vi "BRig_FPGA_v3,91.vi"() -> ()   [LabVIEW 2014]
uses:
  <vilib>/rvi/Emulation/niFpgaGetClockAttributes.vi
  <vilib>/rvi/Emulation/niFpgaSctlEmulationGetInTimedLoop.vi
  <vilib>/rvi/Emulation/niFpgaEmulationReportErrorSimple.vi
  <vilib>/rvi/eio/common/nirviEmuTemplateMethod_errors.vi
  <vilib>/rvi/Emulation/niFpgaCriticalErrorInLSC.vi
  <vilib>/eio/EIONode/EIONode.xnode
panel:
  in  "L2Led_ON":bool
  in  "L1Led_ON":bool
  in  "Rising(F)_or_Falling(T)":bool
  in  "Solenoid_trig_R":bool
  in  "Solenoid_trig_L":bool
  in  "Solenoid_nTotal_R":u32=100
  in  "Solenoid_nTotal_L":u32=100
  in  "L2Led_Baseline":bool
  in  "L1Led_Baseline":bool
  in  "CueLed_Baseline":bool
  in  "I_allReward":bool
  in  "AnaOut_1":u16
  in  "CueLed_Event":bool
  in  "CueLed_nValley":u32=100
  in  "CueLed_nPeak":u32=100
  in  "LC_Event_l2":bool
  in  "LC_Laser_l2":bool
  in  "LC_nShutter_l2":u32=100
  in  "LC_nValley_l2":u32=100
  in  "LC_nPeak_l2":u32=100
  in  "LR_wrong_nDelay_l2":u32
  in  "LR_reward_nDelay_l2":u32
  in  "LR_wrong_nTotal_l2":u32=100
  in  "LR_reward_nTotal_l2":u32=100
  in  "LR_wrong_laser_l2":bool
  in  "LR_wrong_Event_l2":bool
  in  "LR_reward_Laser_l2":bool
  in  "LR_reward_Event_l2":bool
  out "AnaIn_1":u16
  out "AnaIn_0":u16
  out "timeTrial_count":u32
  in  "timeTrial_trig":bool
  in  "k1__counter_per_ms":u16=100 min=100 max=40000 step=1
  in  "LC_nShutter_l1":u32=100
  in  "AnaOut_0":u16
  in  "LC_nValley_l1":u32=100
  in  "LC_nPeak_l1":u32=100
  in  "LC_Event_l1":bool
  in  "LR_wrong_nTotal_l1":u32=100
  in  "LR_wrong_nDelay_l1":u32
  in  "LR_reward_nTotal_l1":u32=100
  in  "LR_reward_nDelay_l1":u32
  in  "LR_reward_Event_l1":bool
  in  "LR_wrong_Event_l1":bool
  out "SelectWrong":bool
  out "SelectReward":bool
  in  "LR_wrong_Laser_l1":bool
  in  "LR_reward_Laser_l1":bool
  in  "Left(F)_or_Right(T)":bool
  in  "ignoreWrong":bool
  in  "SelectionState":bool
  in  "LC_Laser_l1":bool
  in  "FPGA_Stop":bool
  in  "audioTrigger_L":bool
  in  "audioTrigger_R":bool
  in  "audioFreq_L_kHz":u8=14 min=1 max=14 step=1
  in  "audioAmp_L":u16=1 min=1 max=32767 step=1
  in  "audioFreq_R_kHz":u8=14 min=1 max=14 step=1
  in  "audioAmp_R":u16=1 min=1 max=32767 step=1
  in  "A3_SL":bool
  in  "A1_SR":bool
  in  "Counts_Reset":bool
  out "A4_LickR":u32
  out "A2_LickL":u32
  in  "A6_Act":bool
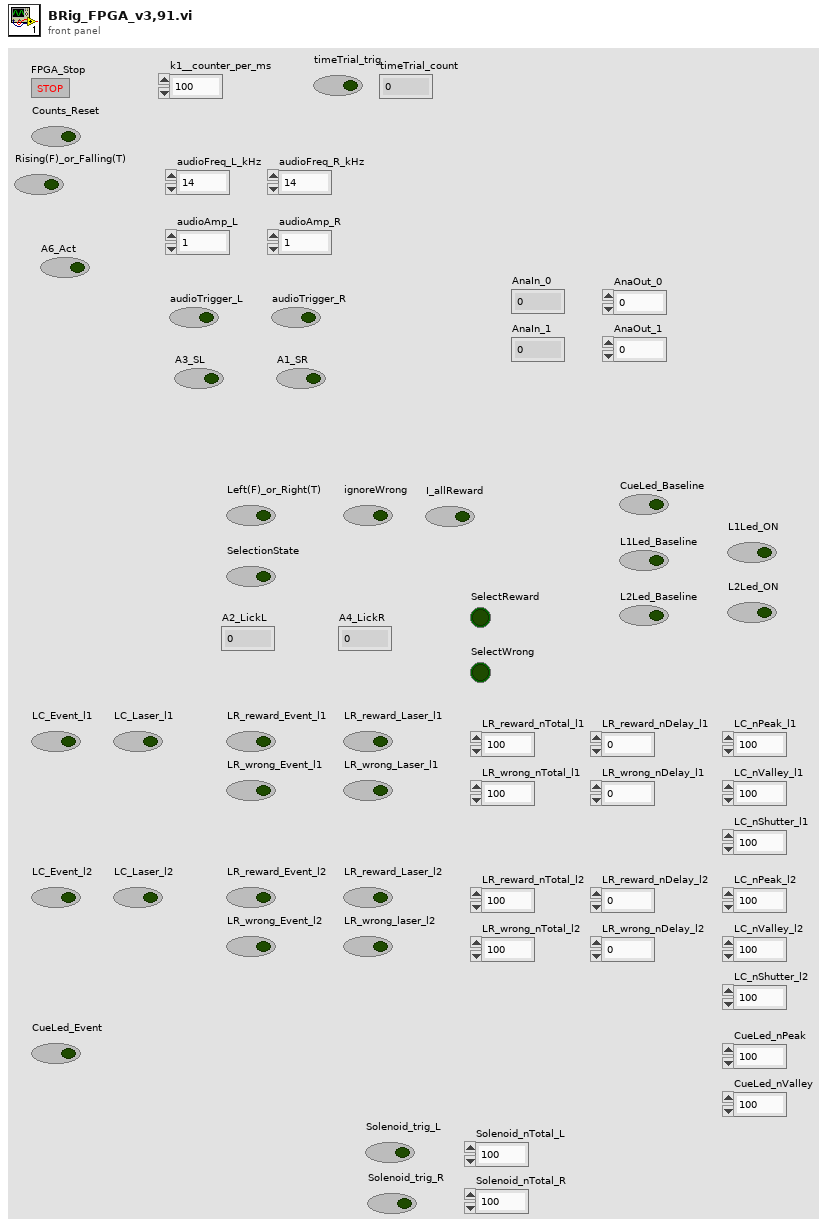
[diagram p1: front panel]
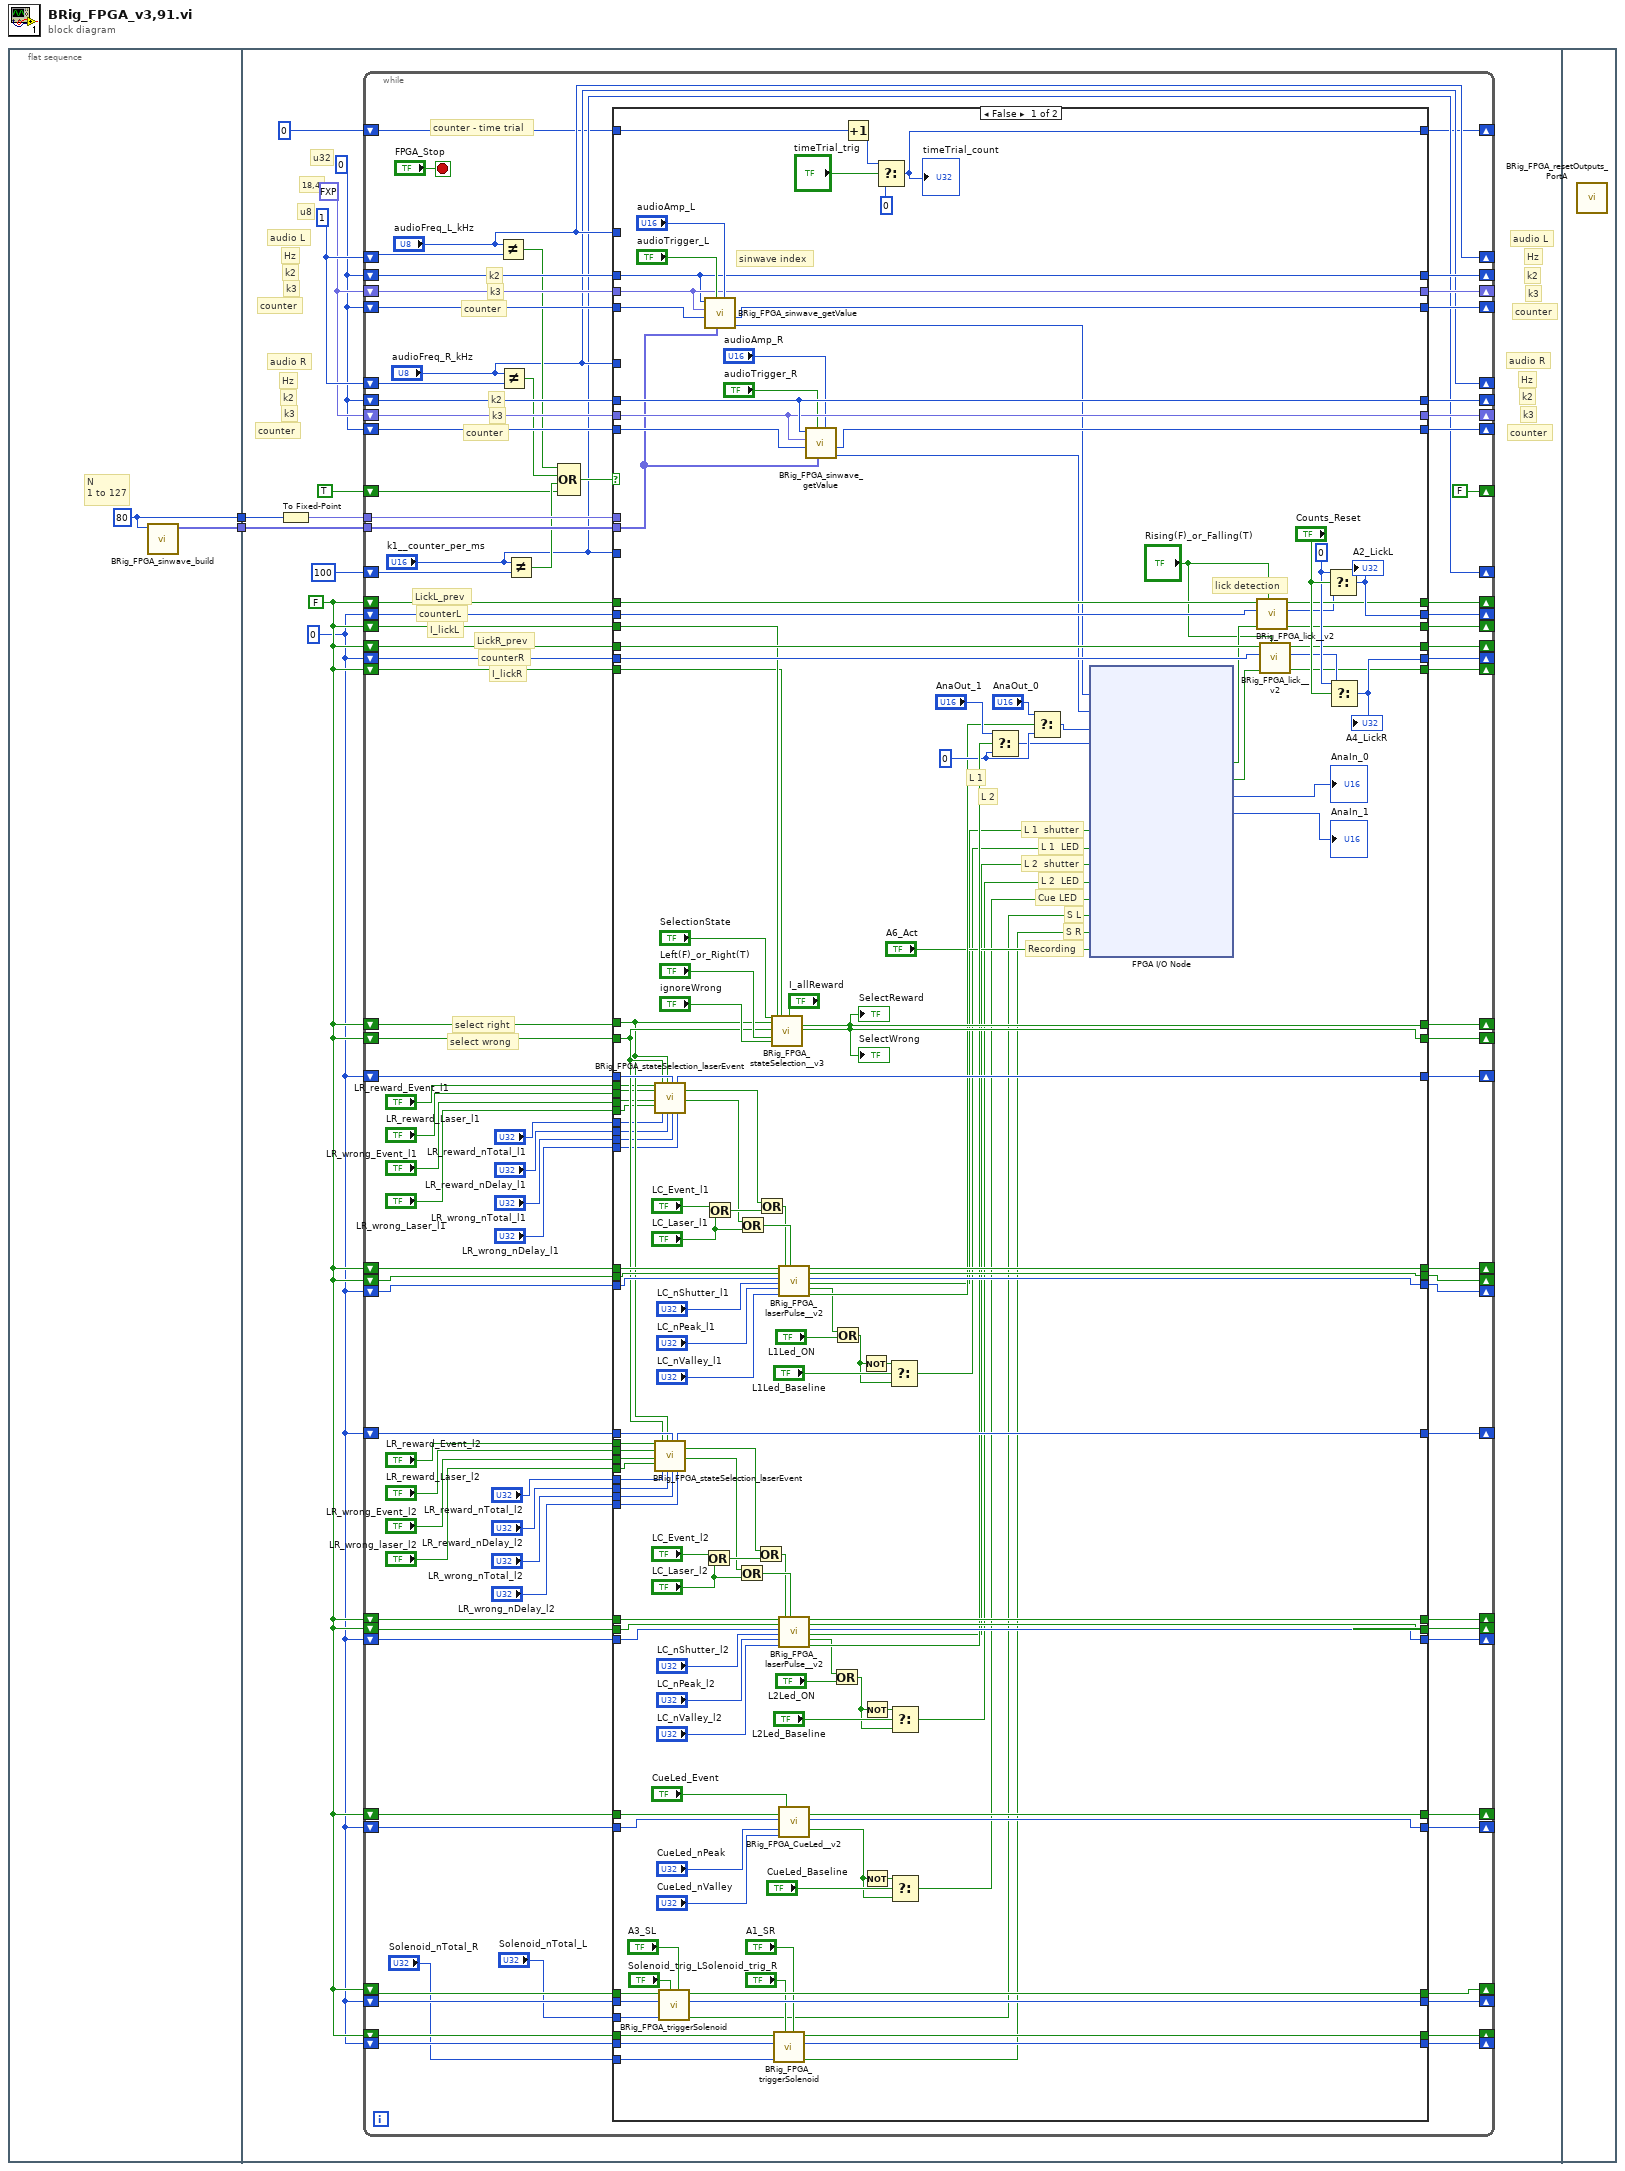
[diagram p0: block diagram]
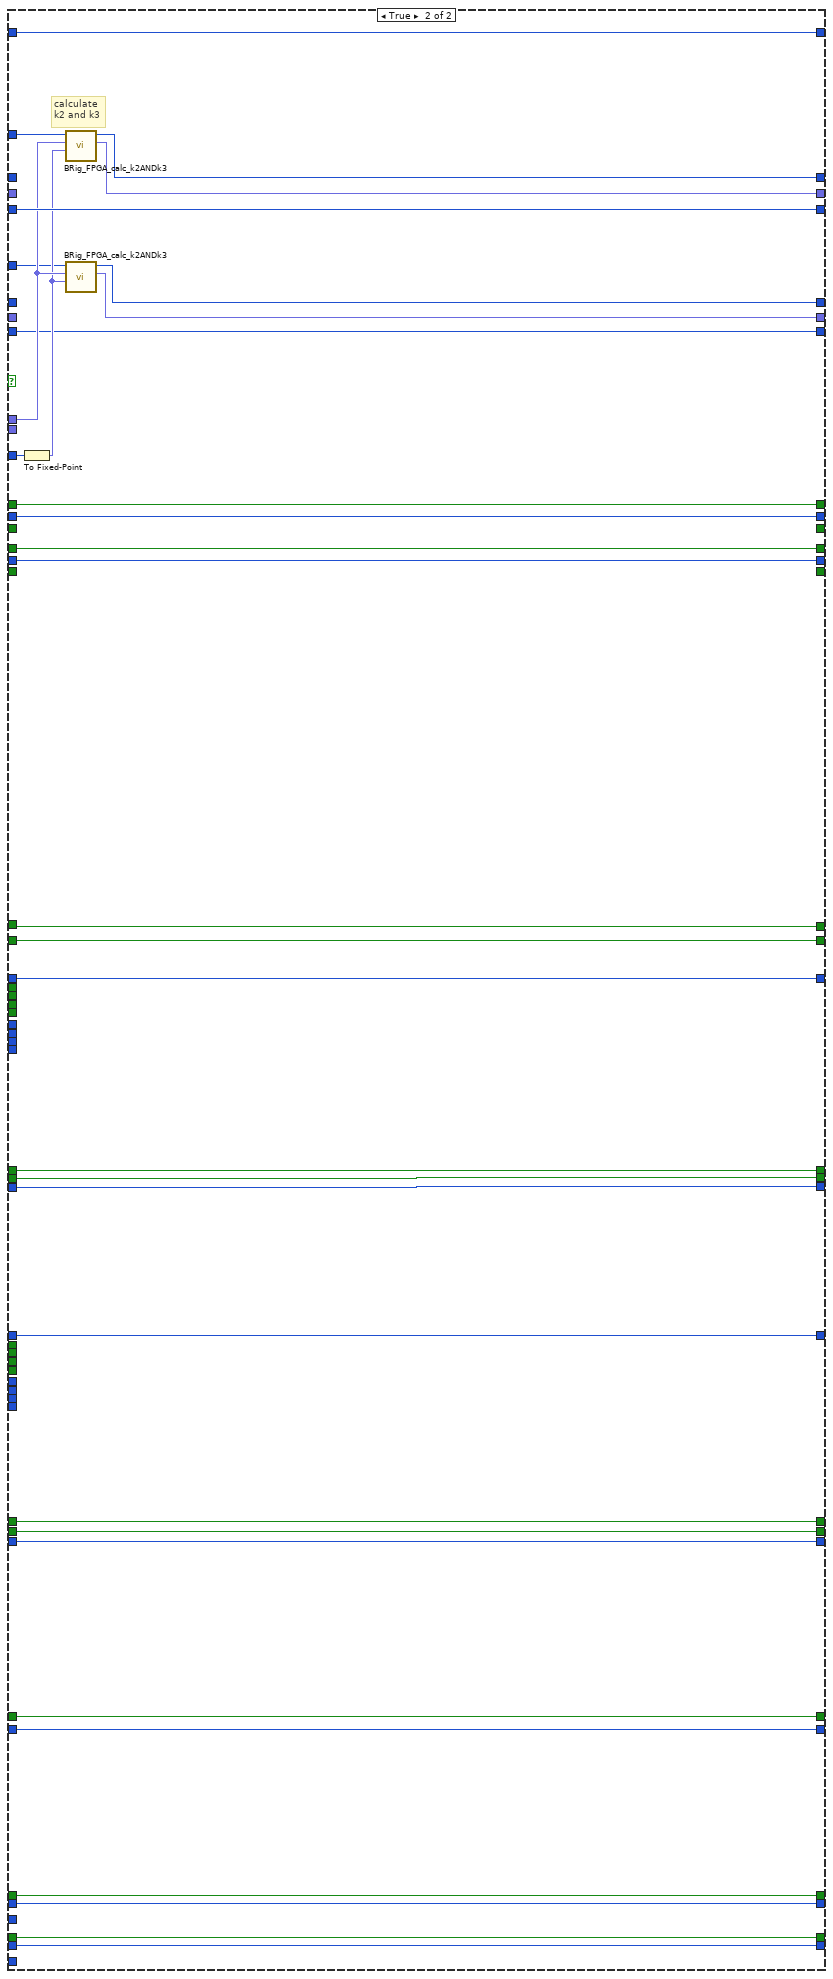
[diagram p2: hidden frame]
diagram:
  n1 = flat-sequence {
    tunnel: [w4] -> w2
    tunnel: [w3] -> w1
    tunnel: w2 -> [w15]
    tunnel: w1 -> [w14]
    frame #0 {
      w3 = 80 ("dimension size")
      # "N\n1 to 127"
      n2 = call "BRig_FPGA_sinwave_build.vi"("input_Npts"=w3) -> ("output_array_sin"=w4:fxp<+/-,16,2>[])  [unwired: 10 in]
    }
    frame #1 {
      w5 = u32 0
      w6 = FALSE
      w10 = u32 0
      w11 = fxp<+,18,4> 0.0
      w12 = u8 1
      # "counter"
      # "k3"
      # "k2"
      # "counter"
      # "k3"
      # "k2"
      # "counter"
      # "counter"
      # "u32"
      # "k3"
      # "k2"
      # "k3"
      # "18,4"
      # "u8"
      # "Hz"
      # "Hz"
      # "audio R"
      # "audio L"
      # "Hz"
      # "k2"
      # "Hz"
      # "audio R"
      # "audio L"
      n3 = To Fixed-Point(number=w14) -> (fixed-point=w13:fxp<+,7,7>)  [unwired: 1 in]
      n4 = while {
        shift-right: ["audioFreq_L_kHz"] -> _
        shift-left: w12 -> [w106]
        shift-right: [w100] -> _
        shift-left: w10 -> [w104]
        shift-right: ["audioFreq_R_kHz"] -> _
        shift-left: w12 -> [w96]
        tunnel: w15 -> [w103]
        tunnel: w13 -> [w102]
        shift-right: [w99] -> _
        shift-left: w11 -> [w101]
        shift-right: [w97] -> _
        shift-left: w10 -> [w98]
        shift-right: [w94] -> _
        shift-left: w10 -> [w95]
        shift-right: [w92] -> _
        shift-left: w11 -> [w93]
        shift-right: [w90] -> _
        shift-left: w10 -> [w91]
        shift-right: ["k1__counter_per_ms"] -> _
        shift-left: u16 100 ("y") -> [w89]
        shift-right: [FALSE] -> _
        shift-left: TRUE -> [w84]
        shift-right: [w77] -> _
        shift-left: w6 -> [w79]
        shift-right: [w76] -> _
        shift-left: w6 -> [w78]
        shift-right: [w74] -> _
        shift-left: w5 -> [w75]
        shift-right: [w72] -> _
        shift-left: w5 -> [w73]
        shift-right: [w69] -> _
        shift-left: w6 -> [w71]
        shift-right: [w68] -> _
        shift-left: w6 -> [w70]
        shift-right: [w66] -> _
        shift-left: w6 -> [w67]
        shift-right: [w64] -> _
        shift-left: w6 -> [w65]
        shift-right: [w62] -> _
        shift-left: u32 0 -> [w63]
        shift-right: [w60] -> _
        shift-left: w5 -> [w61]
        shift-right: [w59] -> _
        shift-left: w6 -> [w56]
        shift-right: [w58] -> _
        shift-left: w6 -> [w55]
        shift-right: [w57] -> _
        shift-left: w5 -> [w54]
        shift-right: [w52] -> _
        shift-left: w5 -> [w53]
        shift-right: [w51] -> _
        shift-left: w6 -> [w48]
        shift-right: [w50] -> _
        shift-left: w6 -> [w47]
        shift-right: [w49] -> _
        shift-left: w5 -> [w46]
        shift-right: [w45] -> _
        shift-left: w6 -> [w43]
        shift-right: [w44] -> _
        shift-left: w5 -> [w42]
        shift-right: [w24] -> _
        shift-left: w5 -> [w25]
        shift-right: [w21] -> _
        shift-left: w6 -> [w23]
        shift-right: [w18] -> _
        shift-left: w6 -> [w20]
        shift-right: [w17] -> _
        shift-left: w5 -> [w19]
        stop <- "FPGA_Stop" stop-if-true
        # "counter"
        # "k3"
        # "k2"
        # "counter"
        # "k3"
        # "k2"
        # "counter - time trial"
        # "I_lickR"
        # "counterR"
        # "LickR_prev"
        # "I_lickL"
        # "counterL"
        # "LickL_prev"
        # "select wrong"
        # "select right"
        n5 = Not Equal?(x="audioFreq_L_kHz", y=w106) -> (x != y?=w88:bool)
        n6 = Not Equal?(x="audioFreq_R_kHz", y=w96) -> (x != y?=w87:bool)
        n7 = Not Equal?(x="k1__counter_per_ms", y=w89) -> (x != y?=w85:bool)
        n8 = Compound Arithmetic op=OR(w88, w87, w85, w84) -> (w86:bool)
        n9 = case shown="False" w86 {
          tunnel: w104 -> [w241 _]
          tunnel: "audioFreq_L_kHz" -> [_ w287]
          tunnel: w103 -> [w234 _]
          tunnel: w102 -> [_ w283]
          tunnel: "k1__counter_per_ms" -> [_ w288]
          tunnel: w101 -> [w242 _]
          tunnel: [w241 w286] -> w100
          tunnel: [w242 w285] -> w99
          tunnel: w98 -> [w246 w284]
          tunnel: [w243 w284] -> w97
          tunnel: w95 -> [w238 _]
          tunnel: [w238 w279] -> w94
          tunnel: w93 -> [w237 _]
          tunnel: [w237 w280] -> w92
          tunnel: w91 -> [w240 w278]
          tunnel: "audioFreq_R_kHz" -> [_ w281]
          tunnel: [w239 w278] -> w90
          tunnel: w79 -> [w229 w277]
          tunnel: w78 -> [w228 w276]
          tunnel: [w233 w277] -> w77
          tunnel: [w226 w276] -> w76
          tunnel: w75 -> [w230 w275]
          tunnel: [w256 w275] -> w74
          tunnel: w73 -> [w227 w274]
          tunnel: [w253 w274] -> w72
          tunnel: w71 -> [w180 w273]
          tunnel: w70 -> [w181 w272]
          tunnel: [w200 w273] -> w69
          tunnel: [w249 w272] -> w68
          tunnel: [w219 w269] -> w59
          tunnel: [w220 w268] -> w58
          tunnel: [w221 w267] -> w57
          tunnel: w67 -> [w223 _]
          tunnel: [w232 _] -> w66
          tunnel: w65 -> [w222 _]
          tunnel: [w224 _] -> w64
          tunnel: w63 -> [w211 w271]
          tunnel: [w208 w271] -> w62
          tunnel: w61 -> [w199 w270]
          tunnel: [w198 w270] -> w60
          tunnel: w56 -> [w197 w269]
          tunnel: w55 -> [w196 w268]
          tunnel: w54 -> [w195 w267]
          tunnel: w53 -> [w183 w266]
          tunnel: [w182 w266] -> w52
          tunnel: [w178 w265] -> w51
          tunnel: [w177 w264] -> w50
          tunnel: [w176 w263] -> w49
          tunnel: w48 -> [w175 w265]
          tunnel: w47 -> [w174 w264]
          tunnel: w46 -> [w173 w263]
          tunnel: [w170 w262] -> w45
          tunnel: [w169 w261] -> w44
          tunnel: w43 -> [w168 w262]
          tunnel: w42 -> [w167 w261]
          tunnel: "LR_reward_Event_l1" -> [w151 _]
          tunnel: "LR_reward_Laser_l1" -> [w150 _]
          tunnel: "LR_wrong_Event_l1" -> [w149 _]
          tunnel: "LR_wrong_Laser_l1" -> [w148 _]
          tunnel: "LR_reward_nTotal_l1" -> [w147 _]
          tunnel: "LR_reward_nDelay_l1" -> [w146 _]
          tunnel: "LR_wrong_nTotal_l1" -> [w145 _]
          tunnel: "LR_wrong_nDelay_l1" -> [w144 _]
          tunnel: "LR_reward_Event_l2" -> [w143 _]
          tunnel: "LR_reward_Laser_l2" -> [w142 _]
          tunnel: "LR_wrong_Event_l2" -> [w141 _]
          tunnel: "LR_wrong_laser_l2" -> [w140 _]
          tunnel: "LR_reward_nTotal_l2" -> [w139 _]
          tunnel: "LR_reward_nDelay_l2" -> [w138 _]
          tunnel: "LR_wrong_nTotal_l2" -> [w137 _]
          tunnel: "LR_wrong_nDelay_l2" -> [w136 _]
          tunnel: w25 -> [w135 w260]
          tunnel: [w130 w260] -> w24
          tunnel: w23 -> [w134 w259]
          tunnel: "Solenoid_nTotal_L" -> [w133 _]
          tunnel: [w129 w259] -> w21
          tunnel: w20 -> [w126 w258]
          tunnel: w19 -> [w125 w257]
          tunnel: [w124 w258] -> w18
          tunnel: [w123 w257] -> w17
          tunnel: "Solenoid_nTotal_R" -> [w122 _]
          frame False {
            w163 = u16 0 ("f")
            w254 = u32 0 ("t")
            # "Cue LED"
            # "L 2  shutter"
            # "L 2  LED"
            # "L 2"
            # "L 1"
            # "L 1  shutter"
            # "L 1  LED"
            # "Recording"
            # "S L"
            # "S R"
            # "sinwave index"
            # "lick detection"
            n10 = call "BRig_FPGA_stateSelection_laserEvent.vi"("I_LR_reward"=w151, "I_LR_reward_laser"=w150, "I_LR_wrong"=w149, "I_LR_wrong_laser"=w148, "I_selectWrong"=w181, "laser_reward_nTotal"=w147, "I_selectReward"=w180, "laser_reward_nDelay"=w146, "counter"=w199, "laser_wrong_nTotal"=w145, "laser_wrong_nDelay"=w144) -> ("output_counter"=w198:u32, "output_I_laserEvent"=w194:bool, "output_I_laserOn"=w193:bool)  [unwired: 6 in]
            n11 = call "BRig_FPGA_stateSelection_laserEvent.vi"("I_LR_reward"=w143, "I_LR_reward_laser"=w142, "I_LR_wrong"=w141, "I_LR_wrong_laser"=w140, "I_selectWrong"=w181, "laser_reward_nTotal"=w139, "I_selectReward"=w180, "laser_reward_nDelay"=w138, "counter"=w183, "laser_wrong_nTotal"=w137, "laser_wrong_nDelay"=w136) -> ("output_counter"=w182:u32, "output_I_laserEvent"=w179:bool, "output_I_laserOn"=w184:bool)  [unwired: 6 in]
            n12 = call "BRig_FPGA_triggerSolenoid.vi"("input_Solenoid_MTrig"="A3_SL", "input_Solenoid_trig"="Solenoid_trig_L", "input_threshold"=w133, "input_counter"=w135, "input_trig"=w134) -> ("output_Solenoid_OnOff"=w119:bool, "output_counter"=w130:u32, "output_trig"=w129:bool)  [unwired: 4 in]
            n13 = Or(x="LC_Event_l2", y="LC_Laser_l2") -> (x .or. y?=w188:bool)
            n14 = call "BRig_FPGA_sinwave_getValue.vi"("audioAmp"="audioAmp_L", "sinwave"=w234, "audioTrigger"="audioTrigger_L", "counter"=w246, "k3"=w242, "k2"=w241) -> ("output_audioValue"=w206:i16, "output_counter"=w243:u32)  [unwired: 4 in]
            n15 = Or(x="LC_Event_l1", y="LC_Laser_l1") -> (x .or. y?=w215:bool)
            n16 = Or(x=w184, y="LC_Laser_l2") -> (x .or. y?=w186:bool)
            n17 = Or(x=w193, y="LC_Laser_l1") -> (x .or. y?=w213:bool)
            n18 = Or(x=w179, y=w188) -> (x .or. y?=w185:bool)
            n19 = Or(x=w194, y=w215) -> (x .or. y?=w212:bool)
            n20 = call "BRig_FPGA_stateSelection__v3.vi"("I_selectionState"="SelectionState", "I_selectRight"=w180, "I_selectWrong"=w181, "I_Left(F)_or_Right(T)"="Left(F)_or_Right(T)", "I_ignoreWrong"="ignoreWrong", "I_lickL"=w223, "I_lickR"=w222, "I_allReward"="I_allReward") -> ("output__I_selectRight"=w200:bool, "output__I_selectWrong"=w249:bool)  [unwired: 18 in]
            "SelectWrong" <- w249
            "SelectReward" <- w200
            n21 = call "BRig_FPGA_triggerSolenoid.vi"("input_Solenoid_MTrig"="A1_SR", "input_Solenoid_trig"="Solenoid_trig_R", "input_threshold"=w122, "input_counter"=w125, "input_trig"=w126) -> ("output_Solenoid_OnOff"=w120:bool, "output_counter"=w123:u32, "output_trig"=w124:bool)  [unwired: 4 in]
            n22 = call "BRig_FPGA_laserPulse__v2.vi"("I_shutter"=w197, "I_peak"=w196, "count"=w195, "laser_Nshutter"="LC_nShutter_l1", "laser_Npeak"="LC_nPeak_l1", "laser_Nvalley"="LC_nValley_l1", "I_laserEvent"=w212, "I_laser"=w213) -> ("output_I_shutter"=w219:bool, "output_I_peak"=w220:bool, "output_count"=w221:u32, "output_shutter"=w115:bool, "output_led"=w111:bool, "output_laser"=w161:bool)  [unwired: 6 in]
            n23 = call "BRig_FPGA_laserPulse__v2.vi"("I_shutter"=w175, "I_peak"=w174, "count"=w173, "laser_Nshutter"="LC_nShutter_l2", "laser_Npeak"="LC_nPeak_l2", "laser_Nvalley"="LC_nValley_l2", "I_laserEvent"=w185, "I_laser"=w186) -> ("output_I_shutter"=w178:bool, "output_I_peak"=w177:bool, "output_count"=w176:u32, "output_shutter"=w117:bool, "output_led"=w108:bool, "output_laser"=w164:bool)  [unwired: 6 in]
            n24 = call "BRig_FPGA_CueLed__v2.vi"("I_peak"=w168, "count"=w167, "laser_Npeak"="CueLed_nPeak", "laser_Nvalley"="CueLed_nValley", "I_CueLed_Event"="CueLed_Event") -> ("output_I_peak"=w170:bool, "output_count"=w169:u32, "output_led"=w156:bool)  [unwired: 12 in]
            n25 = call "BRig_FPGA_sinwave_getValue.vi"("audioAmp"="audioAmp_R", "sinwave"=w234, "audioTrigger"="audioTrigger_R", "counter"=w240, "k3"=w237, "k2"=w238) -> ("output_audioValue"=w205:i16, "output_counter"=w239:u32)  [unwired: 4 in]
            n26 = Or(x=w108, y="L2Led_ON") -> (x .or. y?=w107:bool)
            n27 = Or(x=w111, y="L1Led_ON") -> (x .or. y?=w110:bool)
            n28 = Increment(x=w211) -> (x+1=w210:u32)
            n29 = Not(x=w110) -> (.not. x?=w155:bool)
            n30 = Not(x=w107) -> (.not. x?=w153:bool)
            n31 = Not(x=w156) -> (.not. x?=w158:bool)
            n32 = Select(t=w210, s="timeTrial_trig", f=u32 0) -> (s? t:f=w208:u32)
            "timeTrial_count" <- w208
            n33 = Select(t=w155, s="L1Led_Baseline", f=w110) -> (s? t:f=w114:bool)
            n34 = Select(t=w153, s="L2Led_Baseline", f=w107) -> (s? t:f=w116:bool)
            n35 = Select(t=w158, s="CueLed_Baseline", f=w156) -> (s? t:f=w118:bool)
            n36 = Select(t="AnaOut_1", s=w164, f=w163) -> (s? t:f=w160:u16)
            n37 = Select(t="AnaOut_0", s=w161, f=w163) -> (s? t:f=w165:u16)
            n38 = xnode "FPGA I/O Node"("AudioOut/Left"=w206, "AudioOut/Right"=w205, "ConnectorB/AO0"=w165, "ConnectorB/AO1"=w160, "ConnectorA/DIO6"=w115, "ConnectorB/DIO14"=w114, "ConnectorA/DIO7"=w117, "ConnectorB/DIO15"=w116, "ConnectorB/DIO9"=w118, "ConnectorA/DIO3"=w119, "ConnectorA/DIO5"=w120, "ConnectorA/DIO0"="A6_Act") -> ("ConnectorA/DIO4"=w204:bool, "ConnectorA/DIO2"=w203:bool, "ConnectorB/AI1"=→"AnaIn_0":u16, "ConnectorB/AI2"=→"AnaIn_1":u16)  [unwired: 16 in, 16 out]
            n39 = call "BRig_FPGA_lick__v2.vi"("Rising(F)_or_Falling(T)"="Rising(F)_or_Falling(T)", "I_stateDetector_new"=w204, "counter"=w230, "I_stateDetector_prev"=w229) -> ("output_I_lick"=w232:bool, "output_counter"=w231:u32, "output_I_stateDetector_prev"=w233:bool)  [unwired: 5 in]
            n40 = call "BRig_FPGA_lick__v2.vi"("Rising(F)_or_Falling(T)"="Rising(F)_or_Falling(T)", "I_stateDetector_new"=w203, "counter"=w227, "I_stateDetector_prev"=w228) -> ("output_I_lick"=w224:bool, "output_counter"=w225:u32, "output_I_stateDetector_prev"=w226:bool)  [unwired: 5 in]
            n41 = Select(t=w254, s="Counts_Reset", f=w231) -> (s? t:f=w256:u32)
            "A2_LickL" <- w256
            n42 = Select(t=w254, s="Counts_Reset", f=w225) -> (s? t:f=w253:u32)
            "A4_LickR" <- w253
          }
          frame True {
            # "calculate\nk2 and k3"
            n43 = To Fixed-Point(number=w288) -> (fixed-point=w282:fxp<+,16,16>)  [unwired: 1 in]
            n44 = call "BRig_FPGA_calc_k2ANDk3.vi"("input_k1[count/ms]"=w282, "input_Npts"=w283, "input_freq[kHz]"=w287) -> ("output_k3"=w285:fxp<+,18,4>, "output_k2"=w286:u32)  [unwired: 7 in]
            n45 = call "BRig_FPGA_calc_k2ANDk3.vi"("input_k1[count/ms]"=w282, "input_Npts"=w283, "input_freq[kHz]"=w281) -> ("output_k3"=w280:fxp<+,18,4>, "output_k2"=w279:u32)  [unwired: 7 in]
          }
        }
      }
    }
    frame #2 {
      n46 = call "BRig_FPGA_resetOutputs_PortA.vi"() -> ()  [unwired: 12 in]
    }
  }
